vi "Close.vi"(8 "error in":errorcluster, 11 "ControllerBase in":refnum<class "ControllerBase.lvclass">) -> (0 "error out":errorcluster, 3 "ControllerBase out":refnum<class "ControllerBase.lvclass">)   [LabVIEW 2025, in "ControllerBase.lvclass"]
uses:
  ControllerBase.lvclass
  ControllerBase.lvclass/ControllerBase.ctl
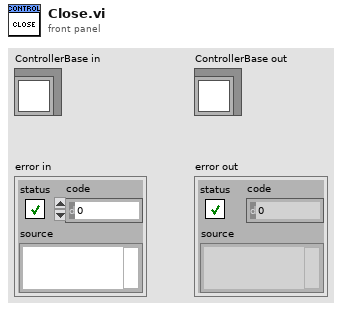
[diagram p1: front panel]
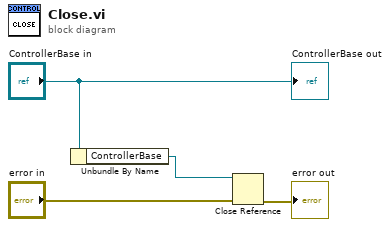
[diagram p0: block diagram]
diagram:
  n1 = Unbundle By Name("ControllerBase in") -> ("ControllerBase"=w1:refnum<k24>)
  n2 = Close Reference(reference=w1, error in (no error)="error in") -> (error out=→"error out":errorcluster)
  "ControllerBase out" <- "ControllerBase in"
